vi "CheckInheritanceEmbedded.vi"(8 "error in (no error)":errorcluster, 10 "Class Path":path, 11 "EmbeddedMainUI in":refnum<class "EmbeddedMainUI.lvclass">) -> (0 "error out":errorcluster, 1 "Embedded SMO?":bool, 2 "Class Path":path, 3 "EmbeddedMainUI out":refnum<class "EmbeddedMainUI.lvclass">)   [LabVIEW 2016, in "EmbeddedMainUI.lvclass"]
uses:
  EmbeddedMainUI.lvclass
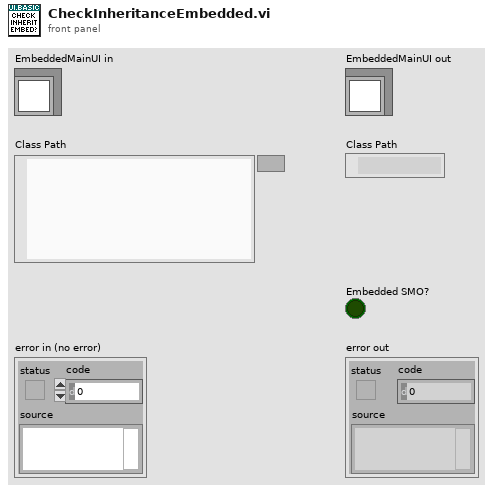
[diagram p1: front panel]
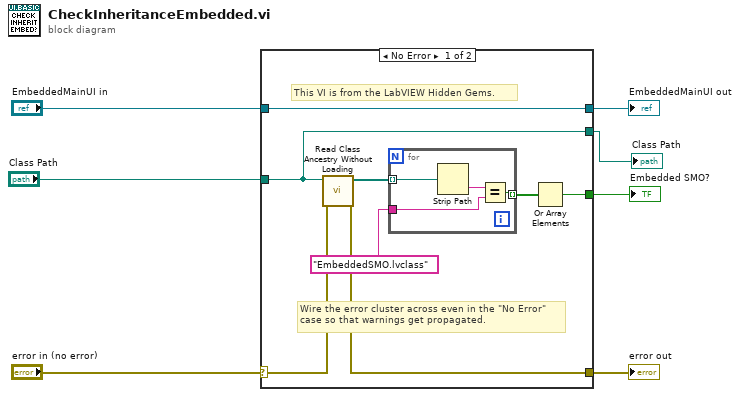
[diagram p0: block diagram]
diagram:
  n1 = case shown="No Error" "error in (no error)" {
    selector: "error in (no error)" -> [w11 w22]
    tunnel: [w10 w22] -> w6
    tunnel: [w15 w21] -> w4
    tunnel: "EmbeddedMainUI in" -> [w15 w21]
    tunnel: "Class Path" -> [w8 w20]
    tunnel: [w9 _] -> w2
    tunnel: [w8 w20] -> w1
    frame No Error {
      # "This VI is from the LabVIEW Hidden Gems."
      # "Wire the error cluster across even in the \"No Error\"\ncase so that warnings get propagated."
      n2 = call <vilib>:"Read Class Ancestry Without Loading.vi"("error in (no error)"=w11, "LabVIEW Class Path"=w8) -> ("error out"=w10:errorcluster, "Class Ancestry"=w14:path[])  [unwired: 8 in]
      n3 = for {
        tunnel: w14 -> [w19] mode=indexing
        tunnel: [w17] -> w13 mode=indexing
        tunnel: "EmbeddedSMO.lvclass" -> [w16]
        n4 = Strip Path(path=w19) -> (name=w18:string)  [unwired: 1 out]
        n5 = Equal?(x=w18, y=w16) -> (x = y?=w17:bool)
      }
      n6 = Or Array Elements(Boolean array=w13) -> (logical OR=w9:bool)
    }
    frame Error {
    }
  }
  "error out" <- w6
  "EmbeddedMainUI out" <- w4
  "Embedded SMO?" <- w2
  "Class Path" <- w1
